vi "GetType.vi"(8 "error in (no error)":errorcluster, 11 "Configure RTD [RTD] Msg":refnum<class "Configure RTD [RTD] Msg.lvclass">) -> (0 "error out":errorcluster, 2 "Data Sample":variant, 3 "Configure RTD [RTD] Msg":refnum<class "Configure RTD [RTD] Msg.lvclass">)   [LabVIEW 2016, in "CS++DMM.lvlib" / "Configure RTD [RTD] Msg.lvclass"]
uses:
  Configure RTD [RTD] Msg.lvclass
  Configure RTD [RTD] Msg.lvclass/Configure RTD [RTD] Msg.ctl
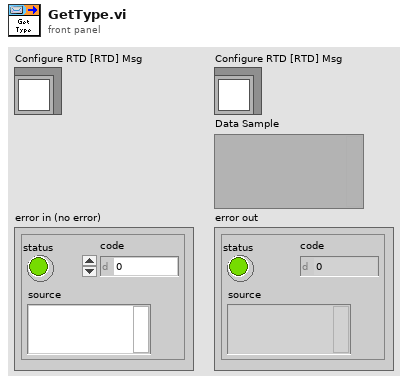
[diagram p1: front panel]
types:
  T1 = cluster{"alpha (0.0)":dbl, "resistance (0.0 ohms)":dbl}
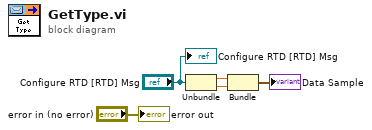
[diagram p0: block diagram]
diagram:
  n1 = Unbundle("Configure RTD [RTD] Msg") -> (w2:dbl, w1:dbl)
  n2 = Bundle("alpha (0.0)"=w2, "resistance (0.0 ohms)"=w1) -> (→"Data Sample":T1)  [unwired: 1 in]
  "error out" <- "error in (no error)"
  "Configure RTD [RTD] Msg" <- "Configure RTD [RTD] Msg"
